vi "MainVI.vi"() -> ()   [LabVIEW 2011]
panel:
  out "Waveform Chart":dbl(graph)
  in  "Numeric":dbl
  in  "stop":bool
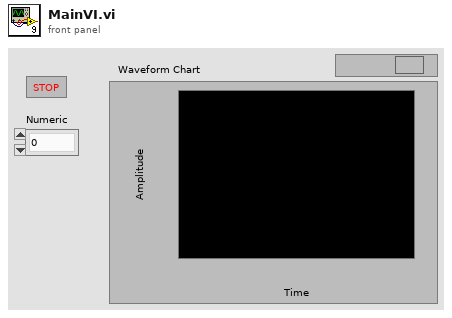
[diagram p1: front panel]
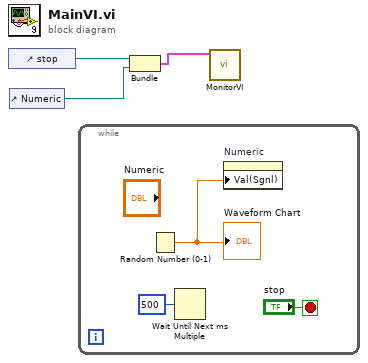
[diagram p0: block diagram]
diagram:
  n1 = control-ref of="stop"() -> (w3:refnum<vi>)
  n2 = control-ref of="Numeric"() -> (w2:refnum<vi>)
  n3 = while {
    stop <- "stop" stop-if-true
    n4 = Random Number (0-1)() -> (number: 0 to 1=w5:dbl)
    "Waveform Chart" <- w5
    n5 = Wait Until Next ms Multiple(millisecond multiple=u32 500) -> ()  [unwired: 1 out]
    n6 = property on="Numeric" class="DigNum (strict)"("Val(Sgnl)"=w5) -> ()  [unwired: 2 in, 2 out]
  }
  n7 = Bundle("stop"=w3, "Numeric"=w2) -> (w1:cluster{"stop":refnum<vi>, "Numeric":refnum<vi>})  [unwired: 1 in]
  n8 = call "MonitorVI.vi"("Input"=w1) -> ()  [unwired: 11 in]
